vi "ChangeTypeInternalVariables.vi"(8 "error in":errorcluster, 11 "ESC Internal Data Structure":T1={"Test_File"="", "Status"="Done", "RF_Center_Freq"="0", "RF_Gain"="0", "BB_Gain"="0", "Error"="", "file_max"="0", "file_index"="0"}) -> (0 "error out":errorcluster, 3 "ESC Internal Data Structure (with types)":T2={"Test_File"=path "", "Status"="Done", "RF_Center_Freq"=0.0, "RF_Gain"=0.0, "BB_Gain"=0.0, "Error 2"="", "file_max"=0, "file_index"=0})   [LabVIEW 2017]
uses:
  TypeDef/ESC Internal Data Structure (types).ctl
  TypeDef/ESC Internal Data Structure (string).ctl
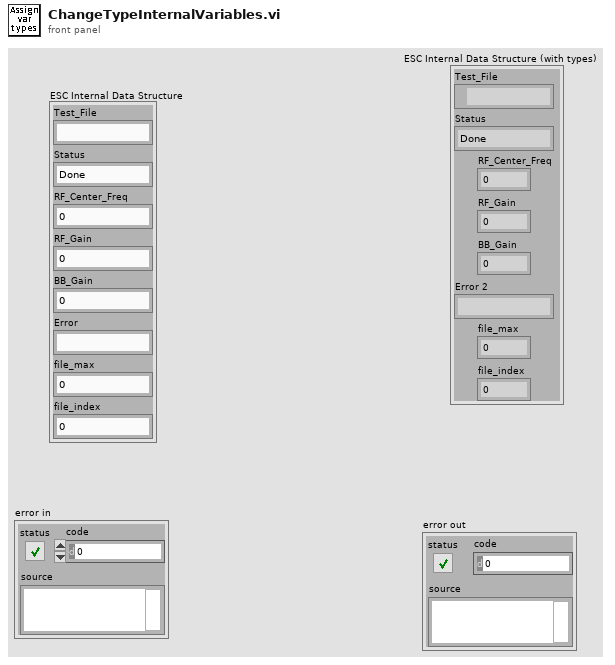
[diagram p1: front panel]
types:
  T1 = typedef "ESC Internal Data Structure (string).ctl" = cluster{"Test_File":string, "Status":string, "RF_Center_Freq":string, "RF_Gain":string, "BB_Gain":string, "Error":string, "file_max":string, "file_index":string}
  T2 = typedef "ESC Internal Data Structure (types).ctl" = cluster{"Test_File":path, "Status":string, "RF_Center_Freq":dbl, "RF_Gain":dbl, "BB_Gain":dbl, "Error 2":string, "file_max":u64, "file_index":u64}
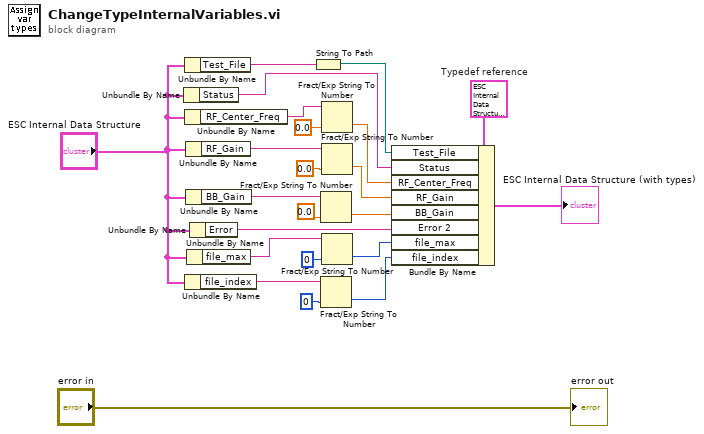
[diagram p0: block diagram]
diagram:
  w19 = T2 {"Test_File"=path "", "Status"="Done", "RF_Center_Freq"=0.0, "RF_Gain"=0.0, "BB_Gain"=0.0, "Error 2"="", "file_max"=0, "file_index"=0}  # Typedef reference
  n1 = Unbundle By Name("ESC Internal Data Structure") -> ("Status"=w13:string)
  n2 = Unbundle By Name("ESC Internal Data Structure") -> ("Test_File"=w22:string)
  n3 = Unbundle By Name("ESC Internal Data Structure") -> ("RF_Center_Freq"=w20:string)
  n4 = Unbundle By Name("ESC Internal Data Structure") -> ("file_index"=w4:string)
  n5 = Unbundle By Name("ESC Internal Data Structure") -> ("RF_Gain"=w23:string)
  n6 = Unbundle By Name("ESC Internal Data Structure") -> ("BB_Gain"=w21:string)
  n7 = Unbundle By Name("ESC Internal Data Structure") -> ("file_max"=w3:string)
  n8 = Unbundle By Name("ESC Internal Data Structure") -> ("Error"=w5:string)
  n9 = String To Path(string=w22) -> (path=w15:path)
  n10 = Fract/Exp String To Number(string=w21, default (0 dbl)=0.0 ("default (0 DBL)")) -> (number=w14:dbl)  [unwired: 2 in, 1 out]
  n11 = Fract/Exp String To Number(string=w4, default (0 dbl)=u64 0 ("default (0 DBL)")) -> (number=w9:u64)  [unwired: 2 in, 1 out]
  n12 = Fract/Exp String To Number(string=w20, default (0 dbl)=0.0 ("default (0 DBL)")) -> (number=w16:dbl)  [unwired: 2 in, 1 out]
  n13 = Fract/Exp String To Number(string=w23, default (0 dbl)=0.0 ("default (0 DBL)")) -> (number=w17:dbl)  [unwired: 2 in, 1 out]
  n14 = Fract/Exp String To Number(string=w3, default (0 dbl)=u64 0 ("default (0 DBL)")) -> (number=w11:u64)  [unwired: 2 in, 1 out]
  n15 = Bundle By Name(cluster=w19, "Test_File"=w15, "Status"=w13, "RF_Center_Freq"=w16, "RF_Gain"=w17, "BB_Gain"=w14, "Error 2"=w5, "file_max"=w11, "file_index"=w9) -> (→"ESC Internal Data Structure (with types)":T2)
  "error out" <- "error in"
